vi "Read Independent Variables.vi"(8 "error in (no error)":errorcluster, 11 "Varian Continuous.lvclass in":refnum<class "Varian Continuous.lvclass">) -> (0 "error out":errorcluster, 1 "size":i32, 2 "Independent Variables":dbl[](array[numeric]), 3 "Varian Continuous.lvclass out":refnum<class "Varian Continuous.lvclass">, 4 "min value":dbl, 5 "max value":dbl)   [LabVIEW 2009, in "Varian Continuous.lvclass"]
doc: "Return the internal array of independent variables for this Scanner, e.g., to write out to a file. Use this method with extreme caution, since it breaks the encapsulation for this class. Do not use it to manipulate a Scanner's internal state."
uses:
  Varian Continuous.lvclass
  Scanner/Scanner.lvclass
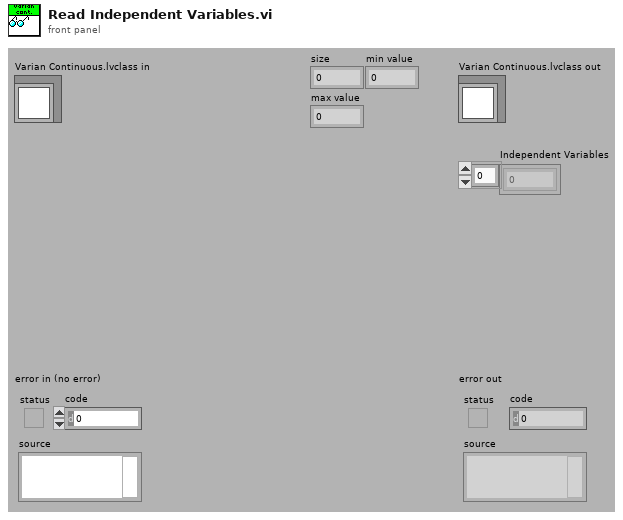
[diagram p1: front panel]
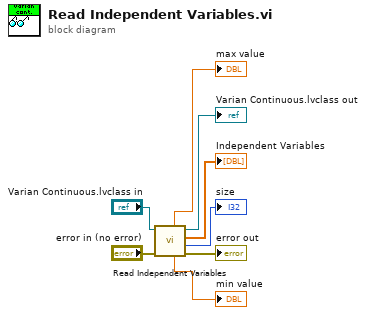
[diagram p0: block diagram]
diagram:
  n1 = call-parent "Read Independent Variables.vi"("error in (no error)"="error in (no error)", "Scanner.lvclass in"="Varian Continuous.lvclass in") -> ("error out"=→"error out":errorcluster, "size"=→"size":i32, "Independent Variables"=→"Independent Variables":dbl[], "Scanner.lvclass out"=→"Varian Continuous.lvclass out":refnum<class "Varian Continuous.lvclass">, "min value"=→"min value":dbl, "max value"=→"max value":dbl)  [unwired: 4 in]
